vi "Main (1).vi"() -> ()   [LabVIEW 2021]
uses:
  Type defs/Current moisteure level.ctl
  Type defs/Lighting Modes.ctl
  Type defs/Solar Position.ctl
  Type defs/Fan STates.ctl
  Type defs/Rain States.ctl
panel:
  out "time":string
  out "Moisture State Machine\nCurrent State":T1
  out "Fan State Machine\n Current State":T2
  out "Tempreture History":i32(graph)
  in  "Time in Hours":u32(knob)=7 min=7 max=19 step=1 scale=7.0..19.0
  out "Solar Panel LCD":T3
  out "Current Light Intensity":i32=6
  in  "Target Light Intensity":u32=5
  out "Light":bool
  in  "Lighting Mode":T4
  out "Current Humidity":i32=6
  out "Dehumidifer ON":bool
  in  "Target Humidity":i32=30
  out "Current Temperature":i32=6
  out "Fan ON":bool
  in  "Target Temperature":i32=50
  out "Current Moisture Level":T5=6
  out "Water Pump ON":bool
  in  "Target Moisture Level":dbl=6.0
  in  "Stop":bool
  out "Dehumidifier":bool
  in  "Soil moisture":u32(slide) scale=0.0..100.0
  in  "LDR":u32(slide) scale=0.0..20.0
  in  "Thermometer":i32(slide) scale=0.0..100.0
  out "Light":bool
  out "Rain":enum32{"No rain", "Rain"}(tab)
  in  "Meter":u32(knob) step=5 scale=0.0..50.0
  out "Fan":enum32{"Fan1", "Fan2", "Fan3", "Fan4"}(tab)
  # "Temperature"
  # "Soil Moisture"
  # "Humidity"
  # "LDRs"
  # "Soil Moisture"
  # "Temperature"
  # "Humidity"
  # "Solar Panel"
  # "Fan"
  # "Lighting Settings"
  # "Water"
  # "Light"
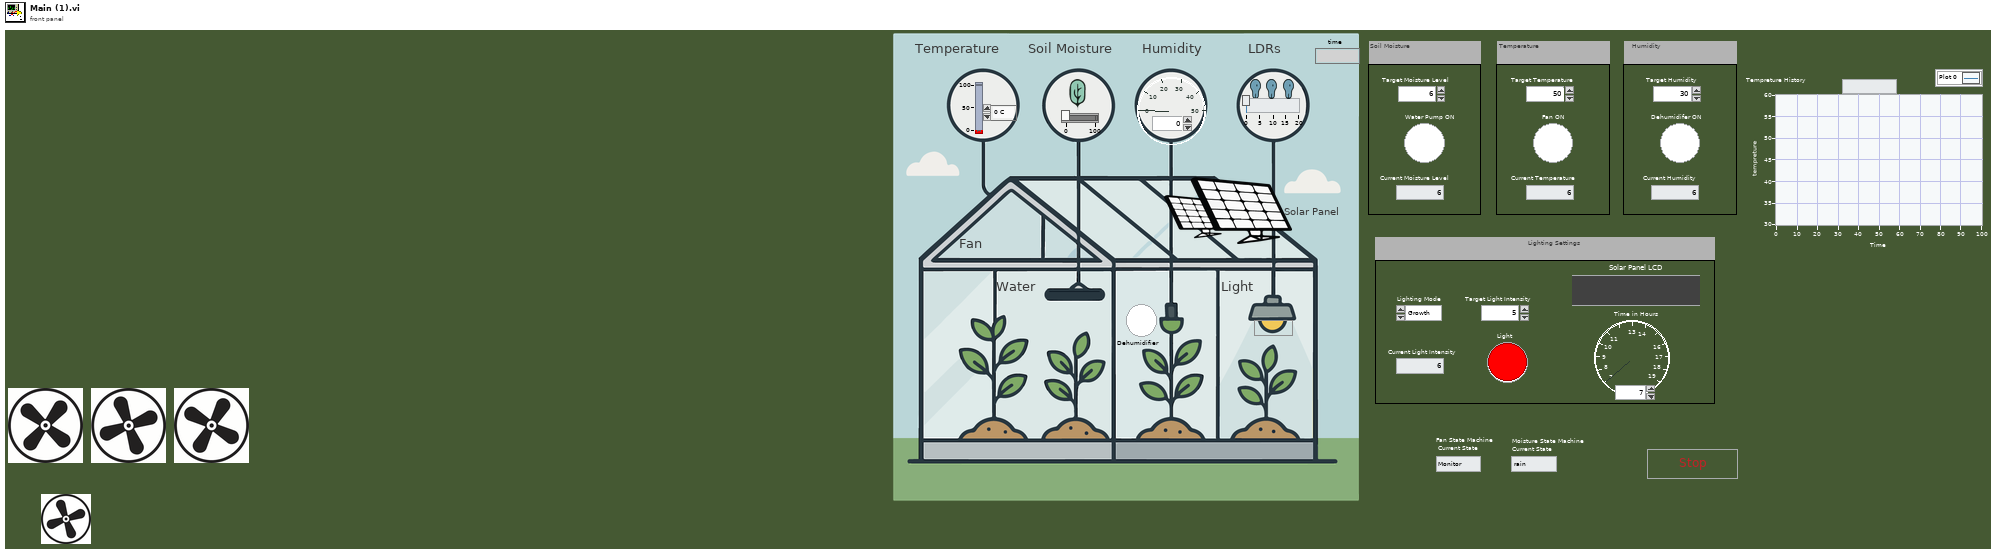
[diagram p1: front panel]
types:
  T1 = typedef "Rain States.ctl" = enum16{"rain", "no rain"}
  T2 = typedef "Fan STates.ctl" = enum16{"Monitor", "Fan On"}
  T3 = typedef "Solar Position.ctl" = string
  T4 = typedef "Lighting Modes.ctl" = enum16{"Growth", "Harvest", "Night"}
  T5 = typedef "Current moisteure level.ctl" = u32
  T6 = cluster{"Tempreture History":i32, "Meter":u32, "Fan ON":bool}
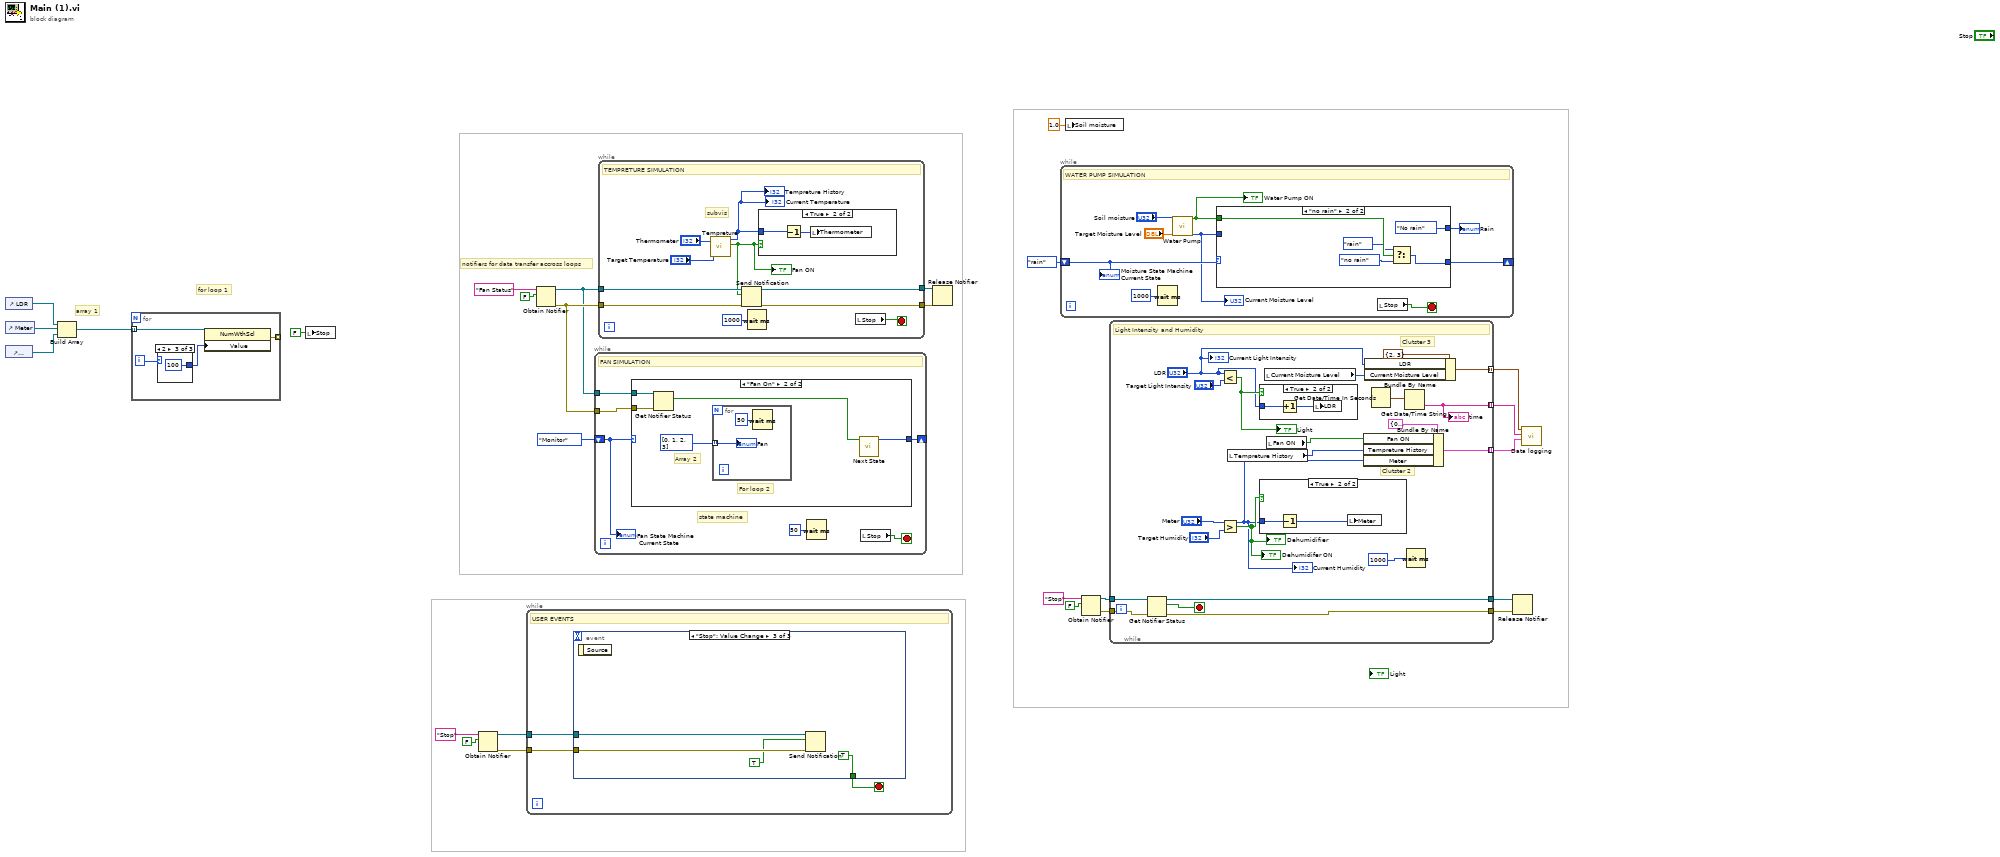
[diagram p0: block diagram]
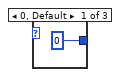
[diagram p2: hidden frame]
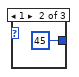
[diagram p3: hidden frame]
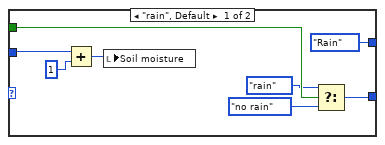
[diagram p4: hidden frame]
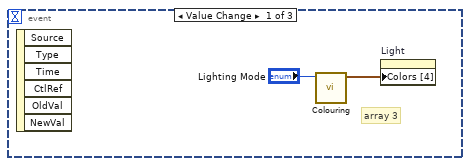
[diagram p5: hidden frame]
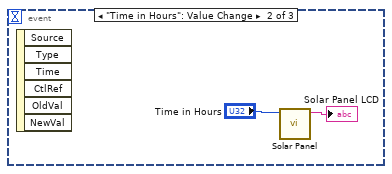
[diagram p6: hidden frame]
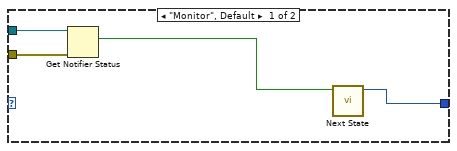
[diagram p9: hidden frame]
diagram:
  # "notifiers for data transfer accross loops"
  # "for loop 1"
  # "array 1"
  n1 = control-ref of="LDR"() -> (w22:refnum<vi>)
  n2 = control-ref of="Meter"() -> (w21:refnum<vi>)
  n3 = control-ref of="Thermometer"() -> (w20:refnum<vi>)
  n4 = Build Array(w22, w21, w20) -> (w23:refnum<vi>[])
  n5 = for {
    tunnel: w23 -> [w30] mode=indexing
    tunnel: [w28] -> _ mode=indexing
    i -> [w31]
    n6 = case shown="2" w31 {
      tunnel: [u32 0 ("LDR") u32 45 ("LDR") u32 100 ("LDR")] -> w29
      frame 0, Default {
      }
      frame 1 {
      }
      frame 2 {
      }
    }
    n7 = property class="NumWthScl"(reference=w30, "Value"=w29) -> (error out=w28:errorcluster)  [unwired: 1 in, 1 out]
  }
  n8 = local write "Stop"(FALSE ("Stop")) -> ()
  n9 = Obtain Notifier(name (unnamed)="Stop", notification data type=FALSE ("Checkbox")) -> (notifier out=w11:refnum<notifier>, error out=w10:errorcluster)  [unwired: 2 in, 1 out]
  n10 = while {
    tunnel: w11 -> [w36]
    tunnel: w10 -> [w35]
    stop <- w37 stop-if-true
    # "USER EVENTS"
    n11 = event shown="[2] \"Stop\": Value Change" {
      selector: _ -> [_ _ _]
      dyn-events: _ -> [_ _ _]
      timeout: _ -> [_ _ _]
      tunnel: [_ _ TRUE] -> w37
      tunnel: w36 -> [_ _ w44]
      tunnel: w35 -> [_ _ w43]
      event Value Change {
        # "array 3"
        n12 = event-data() -> ()  [unwired: 1 in, 6 out]
        n13 = call "Colouring.vi"("Lighting Mode"="Lighting Mode") -> ("Colors [4]"=w39:cluster{"Numeric":u32, "Numeric":u32}[])  [unwired: 10 in]
        n14 = property on="Light" class="Bool (strict)"("Colors [4]"=w39) -> ()  [unwired: 2 in, 2 out]
      }
      event "Time in Hours": Value Change {
        n15 = event-data() -> ()  [unwired: 1 in, 6 out]
        n16 = call "Solar Panel.vi"("Time in Hours"="Time in Hours") -> ("String"=→"Solar Panel LCD":string)  [unwired: 10 in]
      }
      event "Stop": Value Change {
        n17 = event-data() -> ()  [unwired: 1 in, 1 out]
        n18 = Send Notification(notification=TRUE, notifier=w44, error in (no error)=w43) -> ()  [unwired: 2 out]
      }
    }
  }
  n19 = Obtain Notifier(name (unnamed)="Fan Status", notification data type=FALSE ("Checkbox")) -> (notifier out=w14:refnum<notifier>, error out=w15:errorcluster)  [unwired: 2 in, 1 out]
  n20 = while {
    shift-right: [w48] -> _
    shift-left: Fan_STates."Monitor" -> [w49]
    tunnel: w15 -> [w46]
    tunnel: w14 -> [w47]
    stop <- w50 stop-if-true
    # "state machine"
    # "FAN SIMULATION"
    n21 = case shown="\"Fan On\"" w49 {
      tunnel: [w55 w59] -> w48
      tunnel: w47 -> [w54 w58]
      tunnel: w46 -> [w53 w57]
      frame "Monitor", Default {
        n22 = Get Notifier Status(notifier=w54, error in (no error)=w53) -> (current notification=w52:bool)  [unwired: 4 out]
        n23 = call "Next State.vi"("Fan ON"=w52) -> ("s? t:f"=w55:T2)  [unwired: 10 in]
      }
      frame "Fan On" {
        # "Array 2"
        # "For loop 2"
        n24 = Get Notifier Status(notifier=w58, error in (no error)=w57) -> (current notification=w56:bool)  [unwired: 4 out]
        n25 = for {
          tunnel: i32[] [0, 1, 2, 3] -> [w62] mode=indexing
          n26 = Wait (ms)(milliseconds to wait=u32 50) -> ()  [unwired: 1 out]
          "Fan" <- w62
        }
        n27 = call "Next State.vi"("Fan ON"=w56) -> ("s? t:f"=w59:T2)  [unwired: 10 in]
      }
    }
    n28 = Wait (ms)(milliseconds to wait=u32 50) -> ()  [unwired: 1 out]
    n29 = local read "Stop"() -> (w50:bool)
    "Fan State Machine\n Current State" <- w49
  }
  n30 = while {
    tunnel: w14 -> [w68]
    tunnel: w15 -> [w67]
    tunnel: [w65] -> w16
    tunnel: [w64] -> w17
    stop <- w71 stop-if-true
    # "subvis"
    # "TEMPRETURE SIMULATION"
    n31 = call "Tempreture.vi"("Target Temperature"="Target Temperature", "Thermometer  in"="Thermometer") -> ("Checkbox"=w66:bool, "Thermometer  out"=w63:i32)  [unwired: 8 in]
    "Current Temperature" <- w63
    "Fan ON" <- w66
    "Tempreture History" <- w63
    n32 = Send Notification(notification=w66, notifier=w68, error in (no error)=w67) -> (notifier out=w65:refnum<notifier>, error out=w64:errorcluster)
    n33 = Wait (ms)(milliseconds to wait=u32 1000) -> ()  [unwired: 1 out]
    n34 = case shown="True" w66 {
      tunnel: w63 -> [_ w74]
      frame False {
      }
      frame True {
        n35 = Decrement(x=w74) -> (x-1=w73:i32)
        n36 = local write "Thermometer"(w73) -> ()
      }
    }
    n37 = local read "Stop"() -> (w71:bool)
  }
  n38 = Release Notifier(notifier=w16, error in (no error)=w17) -> ()  [unwired: 1 in, 3 out]
  n39 = while {
    shift-right: [w82] -> _
    shift-left: Rain_States."rain" -> [w83]
    stop <- w80 stop-if-true
    # "WATER PUMP SIMULATION"
    n40 = Wait (ms)(milliseconds to wait=u32 1000) -> ()  [unwired: 1 out]
    n41 = call "Water Pump.vi"("Target Moisture Level"="Target Moisture Level", "Soil moisture in"="Soil moisture") -> ("Soil moisture out"=w79:u32, "Checkbox"=w81:bool)  [unwired: 8 in]
    "Water Pump ON" <- w81
    "Current Moisture Level" <- w79
    n42 = case shown="\"no rain\"" w83 {
      tunnel: [w88 w96] -> w82
      tunnel: w81 -> [w87 w95]
      tunnel: w79 -> [w90 _]
      tunnel: [enum32{"No rain", "Rain"}."Rain" ("Rain") enum32{"No rain", "Rain"}."No rain" ("Rain")] -> w78
      frame "rain", Default {
        n43 = Add(x=w90, y=u32 1) -> (x+y=w89:u32)
        n44 = local write "Soil moisture"(w89) -> ()
        n45 = Select(t=Rain_States."rain", s=w87, f=Rain_States."no rain") -> (s? t:f=w88:T1)
      }
      frame "no rain" {
        n46 = Select(t=Rain_States."rain", s=w95, f=Rain_States."no rain") -> (s? t:f=w96:T1)
      }
    }
    "Rain" <- w78
    n47 = local read "Stop"() -> (w80:bool)
    "Moisture State Machine\nCurrent State" <- w83
  }
  n48 = local write "Soil moisture"(1.0 ("Soil moisture")) -> ()
  n49 = Obtain Notifier(name (unnamed)="Stop", notification data type=FALSE ("Checkbox")) -> (notifier out=w7:refnum<notifier>, error out=w6:errorcluster)  [unwired: 2 in, 1 out]
  n50 = while {
    tunnel: w7 -> [w112]
    tunnel: w6 -> [w111]
    tunnel: [w109] -> w4
    tunnel: [w108] -> w5
    tunnel: [w104] -> w3 mode=indexing
    tunnel: [w99] -> w2 mode=indexing
    tunnel: [w97] -> w1 mode=indexing
    stop <- w110 stop-if-true
    # "Clutster 3"
    # "Clutster 2"
    # "Light Intensity and Humidity"
    n51 = Get Notifier Status(notifier=w112, error in (no error)=w111) -> (notifier out=w109:refnum<notifier>, current notification=w110:bool, error out=w108:errorcluster)  [unwired: 2 out]
    n52 = Less?(x="LDR", y="Target Light Intensity") -> (x < y?=w117:bool)
    "Light" <- w117
    n53 = Greater?(x="Meter", y="Target Humidity") -> (0:w114:bool)
    "Dehumidifier" <- w114
    "Dehumidifer ON" <- w114
    n54 = local read "Tempreture History"() -> (w101:i32)
    n55 = case shown="True" w117 {
      tunnel: "LDR" -> [_ w121]
      frame False {
      }
      frame True {
        n56 = Increment(x=w121) -> (x+1=w120:u32)
        n57 = local write "LDR"(w120) -> ()
      }
    }
    n58 = case shown="True" w114 {
      tunnel: "Meter" -> [_ w119]
      frame False {
      }
      frame True {
        n59 = Decrement(x=w119) -> (x-1=w118:u32)
        n60 = local write "Meter"(w118) -> ()
      }
    }
    n61 = local read "Current Moisture Level"() -> (w105:T5)
    n62 = local read "Fan ON"() -> (w102:bool)
    n63 = Bundle By Name(cluster=T6 {"Tempreture History"=0, "Meter"=44, "Fan ON"=TRUE}, "Fan ON"=w102, "Tempreture History"=w101, "Meter"="Meter") -> (w99:T6)
    n64 = Bundle By Name(cluster=cluster{"LDR":u32, "Current Moisture Level":T5} {"LDR"=2, "Current Moisture Level"=3}, "LDR"="LDR", "Current Moisture Level"=w105) -> (w104:cluster{"LDR":u32, "Current Moisture Level":T5})
    n65 = Get Date/Time In Seconds() -> (seconds since 1Jan1904=w98:timestamp)
    n66 = Get Date/Time String(seconds (now)=w98) -> (time string=w97:string)  [unwired: 2 in, 1 out]
    "time" <- w97
    n67 = Wait (ms)(milliseconds to wait=u32 1000) -> ()  [unwired: 1 out]
    "Current Humidity" <- "Meter"
    "Current Light Intensity" <- "LDR"
  }
  n68 = Release Notifier(notifier=w4, error in (no error)=w5) -> ()  [unwired: 1 in, 3 out]
  n69 = call "Data logging.vi"("Array 2"=w2, "Array"=w1, "Array 3"=w3) -> ()  [unwired: 7 in, 2 out]
